vi "test_system_log.vi"() -> ()   [LabVIEW 2019]
uses:
  <vilib>/Utility/SystemLogging/NI_SystemLogging.lvlib
panel:
  in  "severity":i32(ring)=2 items=["Error", "Warning", "Informational"]
  out "error out":errorcluster
  in  "error in":errorcluster
  in  "value":dbl=12.34 format="%#_13g"
  in  "msg_base":string="Test log message"
  # "Use the Windows \"Event Viewer\" to find log messages:\n\"Windows Log\" -> \"Application\"."
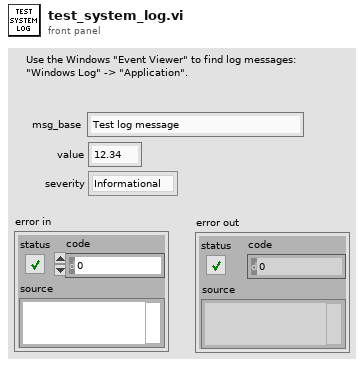
[diagram p1: front panel]
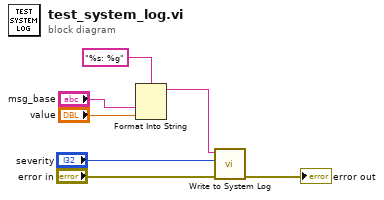
[diagram p0: block diagram]
diagram:
  n1 = Format Into String(format string="%s: %g", "msg_base", "value") -> (resulting string=w2:string)  [unwired: 2 in, 1 out]
  n2 = call <vilib>:"Write to System Log.vi"("error in (no error)"="error in", "severity"="severity", "message"=w2) -> ("error out"=→"error out":errorcluster)  [unwired: 8 in]
